vi "isRunning.vi"(8 "error in (no error)":errorcluster, 11 "ScriptEditorV2 in":refnum<class "ScriptEditorV2.lvclass">) -> (0 "error out":errorcluster, 2 "Running?":bool, 3 "ScriptEditorV2 out":refnum<class "ScriptEditorV2.lvclass">)   [LabVIEW 2011, in "Views.lvlib" / "ScriptEditor.lvlib" / "ScriptEditorV2.lvclass"]
uses:
  ScriptEditorV2.lvclass
  ScriptEditorV2.lvclass/ScriptEditorV2.ctl
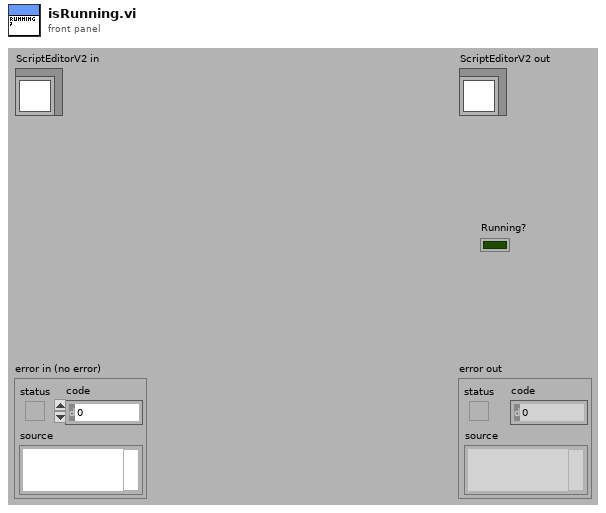
[diagram p1: front panel]
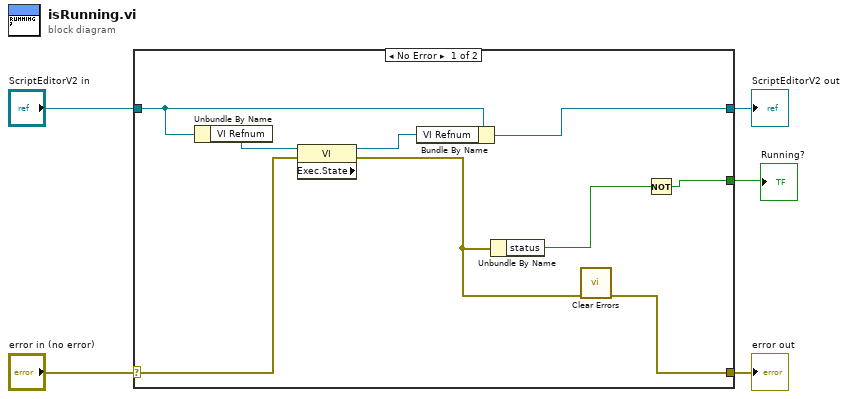
[diagram p0: block diagram]
diagram:
  n1 = case shown="No Error" "error in (no error)" {
    selector: "error in (no error)" -> [w10 w16]
    tunnel: [w6 w16] -> w4
    tunnel: [w11 w15] -> w2
    tunnel: "ScriptEditorV2 in" -> [w12 w15]
    tunnel: [w9 _] -> w1
    frame No Error {
      n2 = Unbundle By Name(w12) -> ("VI Refnum"=w14:refnum<vi>)
      n3 = property class="VI" props=["Exec.State"](reference=w14, error in=w10) -> (reference out=w13:refnum<vi>, error out=w8:errorcluster)  [unwired: 1 out]
      n4 = Bundle By Name(cluster=w12, "VI Refnum"=w13) -> (w11:refnum<class "ScriptEditorV2.lvclass">)
      n5 = Unbundle By Name(w8) -> ("status"=w7:bool)
      n6 = call <vilib>:"Clear Errors.vi"("error in (no error)"=w8) -> ("error out"=w6:errorcluster)  [unwired: 6 in]
      n7 = Not(x=w7) -> (.not. x?=w9:bool)
    }
    frame Error {
    }
  }
  "error out" <- w4
  "ScriptEditorV2 out" <- w2
  "Running?" <- w1
